vi "p2p_distance.vi"(1 "point2":cluster{"X":sgl, "Y":sgl}, 2 "point1":cluster{"X":sgl, "Y":sgl}) -> (0 "poit2poit_dis":dbl)   [LabVIEW 2018]
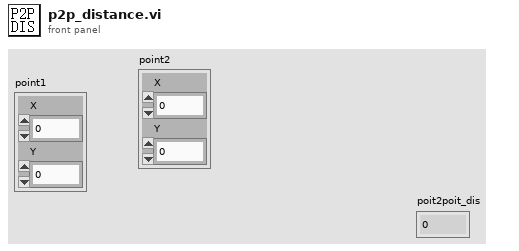
[diagram p1: front panel]
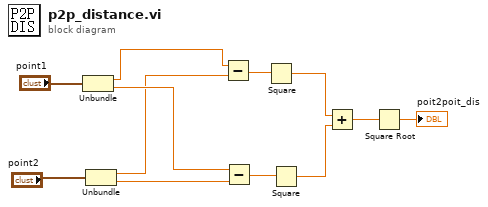
[diagram p0: block diagram]
diagram:
  n1 = Unbundle("point1") -> ("X"=w4:sgl, "Y"=w3:sgl)
  n2 = Unbundle("point2") -> ("X"=w2:sgl, "Y"=w1:sgl)
  n3 = Subtract(x=w4, y=w2) -> (x-y=w10:sgl)
  n4 = Subtract(x=w3, y=w1) -> (x-y=w9:sgl)
  n5 = Square(x=w10) -> (x^2=w8:sgl)
  n6 = Square(x=w9) -> (x^2=w7:sgl)
  n7 = Add(x=w8, y=w7) -> (x+y=w6:sgl)
  n8 = Square Root(x=w6) -> (sqrt(x)=→"poit2poit_dis":sgl)
